vi "Handle.vi"(8 "error in (no error)":errorcluster, 11 "Client_s4gui in":refnum<class "Client_s4gui.lvclass">) -> (0 "error out":errorcluster, 3 "Client_s4gui out":refnum<class "Client_s4gui.lvclass">)   [LabVIEW 2018, in "Client_s4gui.lvclass"]
uses:
  Client_s4gui.lvclass
  Client_s4gui.lvclass/Client_s4gui.ctl
  Client/Client.lvclass
  Comm/Stream/Stream.lvclass
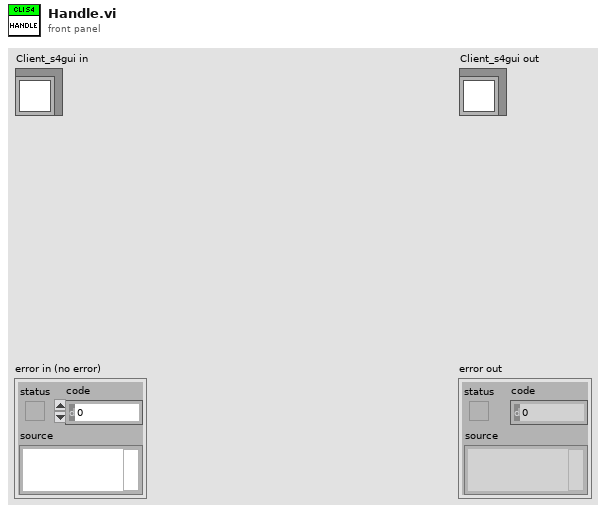
[diagram p1: front panel]
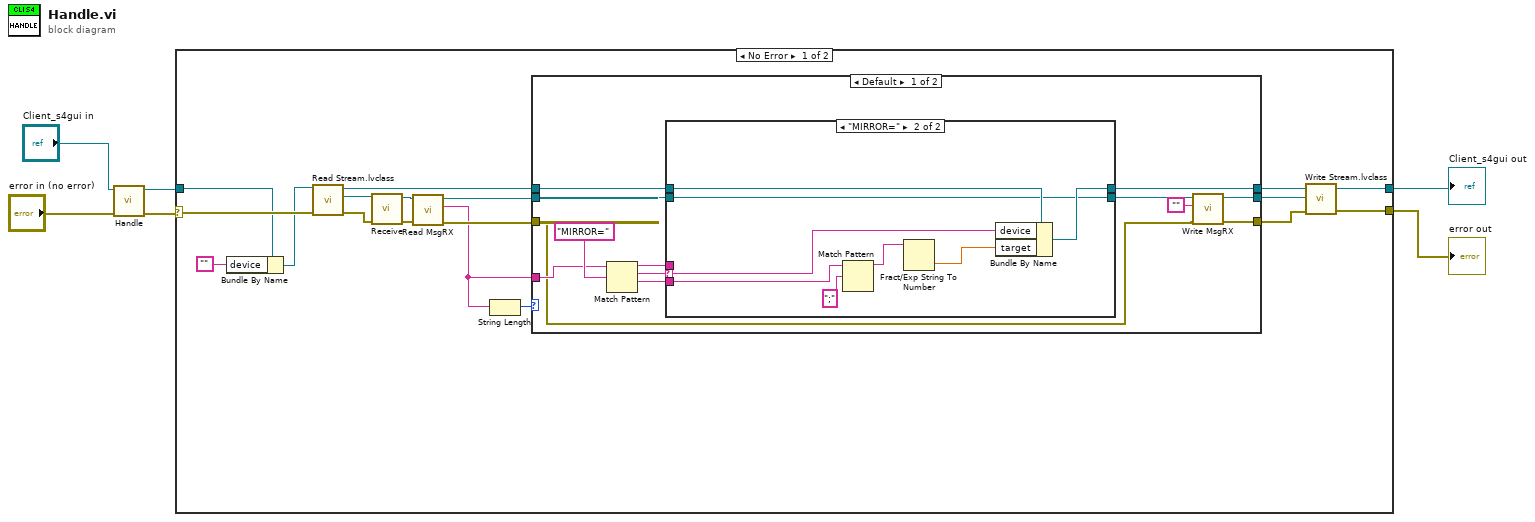
[diagram p0: block diagram]
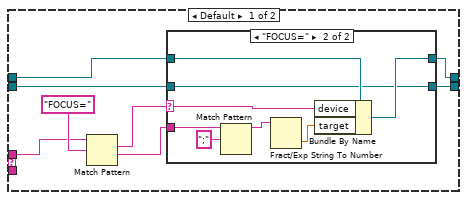
[diagram p2: hidden frame]
diagram:
  n1 = call-parent "Handle.vi"("error in (no error)"="error in (no error)", "Client in"="Client_s4gui in") -> ("error out"=w3:errorcluster, "Client out"=w4:refnum<class "Client_s4gui.lvclass">)  [unwired: 8 in]
  n2 = case shown="No Error" w3 {
    selector: w3 -> [w24 w68]
    tunnel: [w22 w68] -> w1
    tunnel: [w23 w67] -> w2
    tunnel: w4 -> [w9 w67]
    frame No Error {
      n3 = Bundle By Name(cluster=w9, "device"="" ("MsgRX")) -> (w8:refnum<class "Client_s4gui.lvclass">)
      n4 = call-dynamic "Read Stream.lvclass.vi"("error in (no error)"=w24, "Client in"=w8) -> ("error out"=w18:errorcluster, "Stream.lvclass"=w19:refnum<class "Stream.lvclass">, "Client out"=w20:refnum<class "Client_s4gui.lvclass">)  [unwired: 7 in]
      n5 = call-dynamic "Receive.vi"("error in (no error)"=w18, "Stream in"=w19) -> ("error out"=w16:errorcluster, "Stream out"=w17:refnum<class "Stream.lvclass">)  [unwired: 8 in]
      n6 = call-dynamic "Read MsgRX.vi"("error in (no error)"=w16, "Comm in"=w17) -> ("error out"=w13:errorcluster, "MsgRX"=w10:string, "Comm out"=w14:refnum<class "Stream.lvclass">)  [unwired: 7 in]
      n7 = String Length(string=w10) -> (length=w15:i32)
      n8 = case shown="Default" w15 {
        tunnel: [w27 w66] -> w12
        tunnel: [w28 w65] -> w11
        tunnel: w14 -> [w33 w66]
        tunnel: w13 -> [w29 w65]
        tunnel: [w32 w64] -> w21
        tunnel: w20 -> [w34 w64]
        tunnel: w10 -> [w36 _]
        frame Default {
          n9 = Match Pattern(string=w36, regular expression="MIRROR=" ("string")) -> (before substring=w31:string, match substring=w35:string, after substring=w25:string)  [unwired: 1 in, 1 out]
          n10 = case shown="\"MIRROR=\"" w35 {
            selector: w35 -> [_ w57]
            tunnel: w34 -> [w41 w61]
            tunnel: w33 -> [w42 w59]
            tunnel: [w39 w60] -> w32
            tunnel: [w40 w59] -> w30
            tunnel: w31 -> [w38 _]
            tunnel: w25 -> [_ w56]
            frame Default {
              n11 = Match Pattern(string=w38, regular expression="FOCUS=" ("string")) -> (match substring=w44:string, after substring=w43:string)  [unwired: 1 in, 2 out]
              n12 = case shown="\"FOCUS=\"" w44 {
                selector: w44 -> [_ w48]
                tunnel: w43 -> [_ w55]
                tunnel: w41 -> [w46 w52]
                tunnel: w42 -> [w47 w50]
                tunnel: [w46 w51] -> w39
                tunnel: [w47 w50] -> w40
                frame "False", Default {
                }
                frame "FOCUS=" {
                  n13 = Match Pattern(string=w55, regular expression=";") -> (before substring=w53:string)  [unwired: 1 in, 3 out]
                  n14 = Fract/Exp String To Number(string=w53) -> (number=w49:dbl)  [unwired: 3 in, 1 out]
                  n15 = Bundle By Name(cluster=w52, "device"=w48, "target"=w49) -> (w51:refnum<class "Client_s4gui.lvclass">)
                }
              }
            }
            frame "MIRROR=" {
              n16 = Match Pattern(string=w56, regular expression=";") -> (before substring=w62:string)  [unwired: 1 in, 3 out]
              n17 = Fract/Exp String To Number(string=w62) -> (number=w58:dbl)  [unwired: 3 in, 1 out]
              n18 = Bundle By Name(cluster=w61, "device"=w57, "target"=w58) -> (w60:refnum<class "Client_s4gui.lvclass">)
            }
          }
          n19 = call-dynamic "Write MsgRX.vi"("error in (no error)"=w29, "MsgRX"="", "Comm in"=w30) -> ("error out"=w28:errorcluster, "Comm out"=w27:refnum<class "Stream.lvclass">)  [unwired: 7 in]
        }
        frame 0 {
        }
      }
      n20 = call-dynamic "Write Stream.lvclass.vi"("error in (no error)"=w11, "Stream.lvclass"=w12, "Client in"=w21) -> ("error out"=w22:errorcluster, "Client out"=w23:refnum<class "Client_s4gui.lvclass">)  [unwired: 7 in]
    }
    frame Error {
    }
  }
  "error out" <- w1
  "Client_s4gui out" <- w2
